vi "Calc Rotation Value.vi"(1 "PID gains":T1={"proportional gain (Kc)"=1.0, "integral time (Ti, min)"=0.01, "derivative time (Td, min)"=0.0} {"derivative time (Td, min)" format="%.3f"; "integral time (Ti, min)" format="%.3f"; "proportional gain (Kc)" format="%.3f"}, 2 "Gyro Angle":dbl, 3 "Joystick Rotation":dbl, 4 "Rotation Data":T2) -> (0 "Rotation Value":dbl)   [LabVIEW 2018]
uses:
  Controls/DriveJoystickButtonMapping.ctl
  <vilib>/addons/control/pid/pid.llb/PID (DBL).vi
  <vilib>/addons/control/pid/NI_PID_pid.lvlib
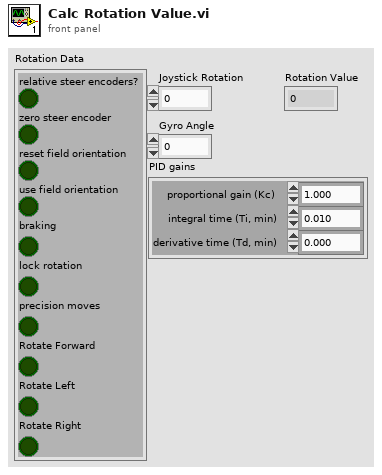
[diagram p1: front panel]
types:
  T1 = cluster{"proportional gain (Kc)":dbl, "integral time (Ti, min)":dbl, "derivative time (Td, min)":dbl}
  T2 = typedef "DriveJoystickButtonMapping.ctl" = cluster{"relative steer encoders?":bool, "zero steer encoder":bool, "reset field orientation":bool, "use field orientation":bool, "braking":bool, "lock rotation":bool, "precision moves":bool, "Rotate Forward":bool, "Rotate Left":bool, "Rotate Right":bool}
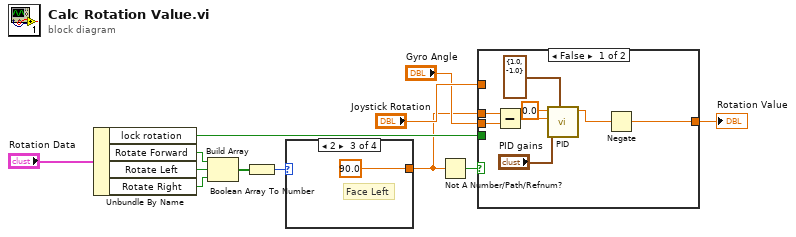
[diagram p0: block diagram]
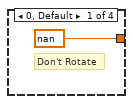
[diagram p2: hidden frame]
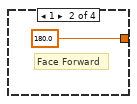
[diagram p3: hidden frame]
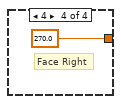
[diagram p4: hidden frame]
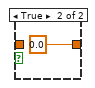
[diagram p6: hidden frame]
diagram:
  n1 = Unbundle By Name("Rotation Data") -> ("lock rotation"=w10:bool, "Rotate Forward"=w6:bool, "Rotate Left"=w5:bool, "Rotate Right"=w4:bool)
  n2 = Build Array(w6, w5, w4) -> (w7:bool[])
  n3 = Boolean Array To Number(Boolean array=w7) -> (number=w8:u32)
  n4 = case shown="2" w8 {
    tunnel: [nan 180.0 90.0 270.0] -> w1
    frame 0, Default {
      # "Don't Rotate"
    }
    frame 1 {
      # "Face Forward"
    }
    frame 2 {
      # "Face Left"
    }
    frame 4 {
      # "Face Right"
    }
  }
  n5 = Not A Number/Path/Refnum?(number/path/refnum=w1) -> (NaN/Path/Refnum?=w3:bool)
  n6 = case shown="False" w3 {
    tunnel: "Joystick Rotation" -> [_ w25]
    tunnel: w10 -> [_ w27]
    tunnel: [w17 w26] -> w9
    tunnel: "Gyro Angle" -> [w24 _]
    tunnel: w1 -> [w23 _]
    frame False {
      n7 = Subtract(x=w23, y=w24) -> (x-y=w22:dbl)
      n8 = call-poly <vilib>:"PID.vi"("output range"=cluster{"output high":dbl, "output low":dbl} {"output high"=1.0, "output low"=-1.0}, "PID gains"="PID gains", "process variable"=w22, "setpoint"=0.0) -> ("output"=w18:dbl)  [unwired: 6 in, 1 out]
      n9 = Negate(x=w18) -> (-x=w17:dbl)
    }
    frame True {
      n10 = case shown="False" w27 {
        tunnel: [w28 0.0] -> w26
        tunnel: w25 -> [w28 _]
        frame False {
        }
        frame True {
        }
      }
    }
  }
  "Rotation Value" <- w9
